vi "Control Parameters Status.vi"(0 "VISA resource name":refnum<visa-resource-name>, 5 "Loop (1:Loop 1)":u16(ring)=1 items=["Loop 1"=1, "Loop 2"=2], 11 "error in (no error)":errorcluster) -> (2 "Heater Range":u16(ring) items=["Off", "Low (loop 1) or On (loop 2)", "High (loop 1)"], 3 "Heater Resistance":u16(ring)=1 items=["25 Ohm"=1, "50 Ohm"=2], 4 "VISA resource name out":refnum<visa-resource-name>, 6 "Gain (P)":dbl format="%.1f", 8 "Reset (I)":dbl format="%.1f", 10 "Rate (D)":u16, 13 "Tuning Active":bool, 14 "Manual Heater Power":dbl format="%.3f", 15 "error out":errorcluster)   [LabVIEW 2019, in "Lake Shore 325.lvlib"]
doc: "This VI returns control parameters - PID, Manual Heater Output, Heater Range, Heater Resistance, and Tuning Status."
uses:
  Lake Shore 325.lvlib
  Instance           1 33Saved   Control Parameters Status .vi
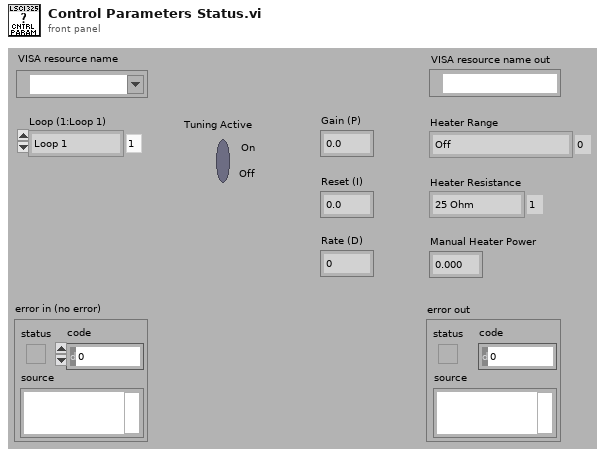
[diagram p1: front panel]
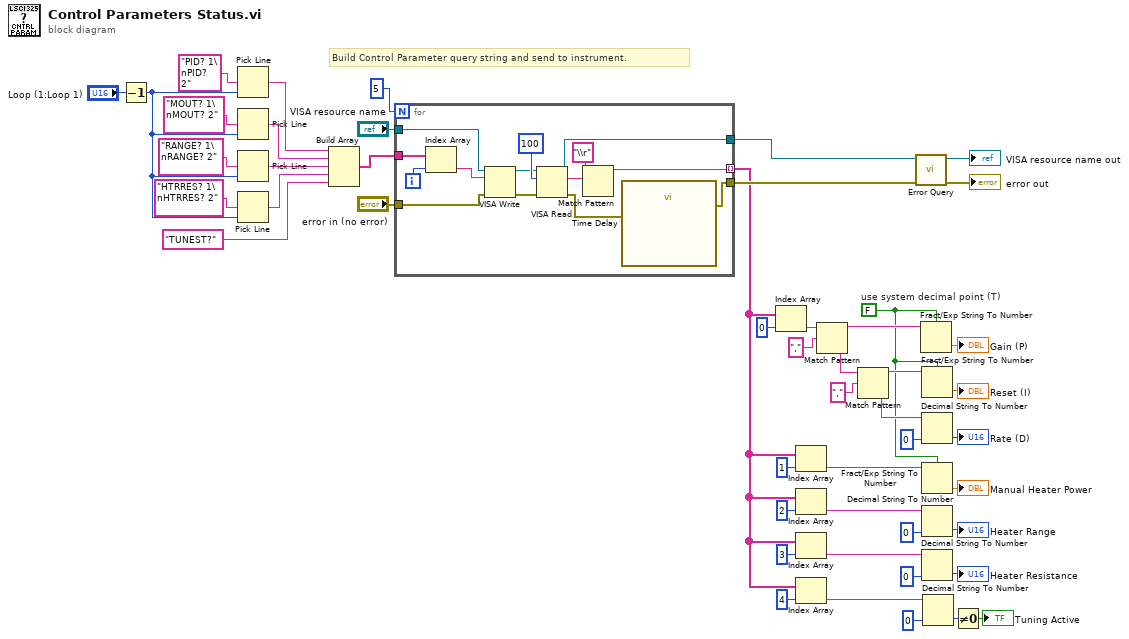
[diagram p0: block diagram]
diagram:
  w1 = FALSE  # use system decimal point (T)
  # "Build Control Parameter query string and send to instrument."
  n1 = Decrement(x="Loop (1:Loop 1)") -> (x-1=w2:u16)
  n2 = Pick Line(multi-line string="PID? 1\nPID? 2", line index=w2) -> (output string=w40:string)  [unwired: 1 in]
  n3 = Pick Line(multi-line string="MOUT? 1\nMOUT? 2", line index=w2) -> (output string=w38:string)  [unwired: 1 in]
  n4 = Pick Line(multi-line string="RANGE? 1\nRANGE? 2", line index=w2) -> (output string=w37:string)  [unwired: 1 in]
  n5 = Pick Line(multi-line string="HTRRES? 1\nHTRRES? 2", line index=w2) -> (output string=w33:string)  [unwired: 1 in]
  n6 = Build Array(w40, w38, w37, w33, "TUNEST?") -> (w45:string[])
  n7 = for {
    N: 5 -> [_]
    tunnel: [w56] -> w44
    tunnel: [w51] -> w43
    tunnel: "VISA resource name" -> [w55]
    tunnel: "error in (no error)" -> [w54]
    tunnel: w45 -> [w53]
    tunnel: [w52] -> w15 mode=indexing
    i -> [w58]
    n8 = Index Array(array=w53, index=w58) -> (element=w57:string)
    n9 = VISA Write(VISA resource name=w55, write buffer=w57, error in (no error)=w54) -> (VISA resource name out=w60:refnum<visa-resource-name>, error out=w59:errorcluster)  [unwired: 1 out]
    n10 = VISA Read(VISA resource name=w60, byte count=100, error in (no error)=w59) -> (VISA resource name out=w56:refnum<visa-resource-name>, read buffer=w62:string, error out=w50:errorcluster)  [unwired: 1 out]
    n11 = Match Pattern(string=w62, regular expression="\\r") -> (before substring=w52:string)  [unwired: 1 in, 3 out]
    n12 = call "Time Delay"("error in (no error)"=w50) -> ("error out"=w51:errorcluster)  [unwired: 10 in]
  }
  n13 = Index Array(array=w15, index=0) -> (element=w28:string)
  n14 = Index Array(array=w15, index=1) -> (element=w14:string)
  n15 = Index Array(array=w15, index=2) -> (element=w11:string)
  n16 = Index Array(array=w15, index=3) -> (element=w8:string)
  n17 = Index Array(array=w15, index=4) -> (element=w4:string)
  n18 = Match Pattern(string=w28, regular expression=",") -> (before substring=w24:string, after substring=w26:string)  [unwired: 1 in, 2 out]
  n19 = Match Pattern(string=w26, regular expression=",") -> (before substring=w23:string, after substring=w22:string)  [unwired: 1 in, 2 out]
  n20 = call "Error Query.vi"("error in (no error)"=w43, "VISA resource name"=w44) -> ("error out"=→"error out":errorcluster, "VISA resource name out"=→"VISA resource name out":refnum<visa-resource-name>)  [unwired: 7 in, 1 out]
  n21 = Fract/Exp String To Number(use system decimal point (T)=w1, string=w24) -> (number=→"Gain (P)":dbl)  [unwired: 2 in, 1 out]
  n22 = Fract/Exp String To Number(use system decimal point (T)=w1, string=w23) -> (number=→"Reset (I)":dbl)  [unwired: 2 in, 1 out]
  n23 = Decimal String To Number(string=w22, default (0L)=0) -> (number=→"Rate (D)":i32)  [unwired: 1 in, 1 out]
  n24 = Fract/Exp String To Number(use system decimal point (T)=w1, string=w14) -> (number=→"Manual Heater Power":dbl)  [unwired: 2 in, 1 out]
  n25 = Decimal String To Number(string=w11, default (0L)=0) -> (number=→"Heater Range":i32)  [unwired: 1 in, 1 out]
  n26 = Decimal String To Number(string=w8, default (0L)=0) -> (number=→"Heater Resistance":i32)  [unwired: 1 in, 1 out]
  n27 = Decimal String To Number(string=w4, default (0L)=u16 0) -> (number=w5:u16)  [unwired: 1 in, 1 out]
  n28 = Not Equal To 0?(x=w5) -> (x != 0?=→"Tuning Active":bool)
